vi "Min_Max_function.vi"() -> ()   [LabVIEW 2019]
panel:
  out "min(x,y)":u8
  out "max(x,y)":u8
  in  "Numeric 2":u8
  in  "Numeric":u8
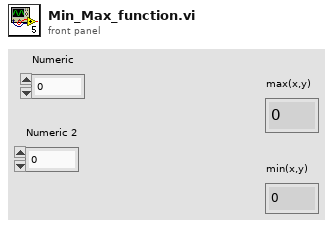
[diagram p1: front panel]
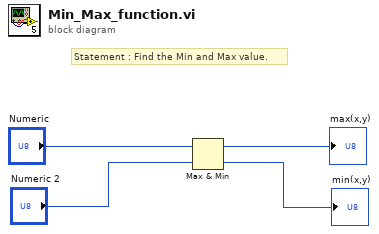
[diagram p0: block diagram]
diagram:
  # "Statement : Find the Min and Max value."
  n1 = Max & Min(x="Numeric", y="Numeric 2") -> (max(x,y)=→"max(x,y)":u8, min(x,y)=→"min(x,y)":u8)
